vi "scan2D.vi"() -> ()   [LabVIEW 2019]
uses:
  National Instruments/LabVIEW 2019/instr.lib/Stanford Research 830/Public/Data/Read (All Parameters).vi
  National Instruments/LabVIEW 2019/instr.lib/Stanford Research 830/Stanford Research 830.lvlib
panel:
  in  "stop":bool
  in  "Tab Control":enum32{"Page 1", "Page 2", "Page 3"}(tab)
  out "progress":u8(slide) scale=0.0..100.0
  in  "Set zero":bool
  in  "Scanning range":T1
  in  "wait time":u32=3000
  in  "start":bool
  in  "file path (use dialog)":path
  in  "Cluster 2":T2={"Input Connection (0: Single-Ended Voltage) "=2, "Input Coupling (0: AC)"=0, "Input Notch Filter (0: None)"=0, "Input Shield Grounding (0: Float)"=1, "Internal Reference Frequency (1000 Hz)"=200.0, "Dynamic Reserve (-1: Auto Reserve)"=2, "Sensitivity (-1: Auto gain)"=16, "Time Constant (8: 100ms)"=10, "Low Pass Filter Slope (1: 12dB/oct)"=3, "Enable Sync Filter (F: Disable)"=FALSE, "save"=FALSE} {"Low Pass Filter Slope (1: 12dB/oct)" items=["6 dB/oct", "12 dB/oct", "18 db/oct", "24 dB/oct"]; "Time Constant (8: 100ms)" items=["10 us", "30 us", "100 us", "300 us", "1 ms", "3 ms", "10 ms", "30 ms", "100 ms", "300 ms", "1 s", "3 s", "10 s", "30 s", "100 s", "300 s", "1 ks", "3 ks", "10 ks", "30 ks"]; "Sensitivity (-1: Auto gain)" items=["Auto Gain"=-1, "2 nV/fA"=0, "5 nV/fA"=1, "10 nV/fA"=2, "20 nV/fA"=3, "50 nV/fA"=4, "100 nV/fA"=5, "200 nV/fA"=6, "500 nV/fA"=7, "1 uV/pA"=8, "2 uV/pA"=9, "5 uV/pA"=10, "10 uV/pA"=11, "20 uV/pA"=12, "50 uV/pA"=13, "100 uV/pA"=14, "200 uV/pA"=15, "500 uV/pA"=16, "1 mV/nA"=17, "2 mV/nA"=18, "5 mV/nA"=19, "10 mV/nA"=20, "20 mV/nA"=21, "50 mV/nA"=22, "100 mV/nA"=23, "200 mV/nA"=24, "500 mV/mA"=25, "1 V/uA"=26]; "Dynamic Reserve (-1: Auto Reserve)" items=["Auto Reserve"=-1, "High Reserve"=0, "Normal"=1, "Low Noise"=2]; "Input Shield Grounding (0: Float)" items=["Float", "Ground"]; "Input Notch Filter (0: None)" items=["None", "Line Notch", "2x Line Notch", "Both Notch Filters"]; "Input Coupling (0: AC)" items=["AC", "DC"]; "Input Connection (0: Single-Ended Voltage)" items=["Single-Ended Voltage", "Differential Voltage", "1 MOhm Current Gain", "100 MOhm Current Gain"]}
  in  "VISA resource name":refnum<visa-resource-name>="GPIB0::8::INSTR"
  out "error out":errorcluster
  out "Intensity Graph":dbl[][](graph)
  # "All relative position"
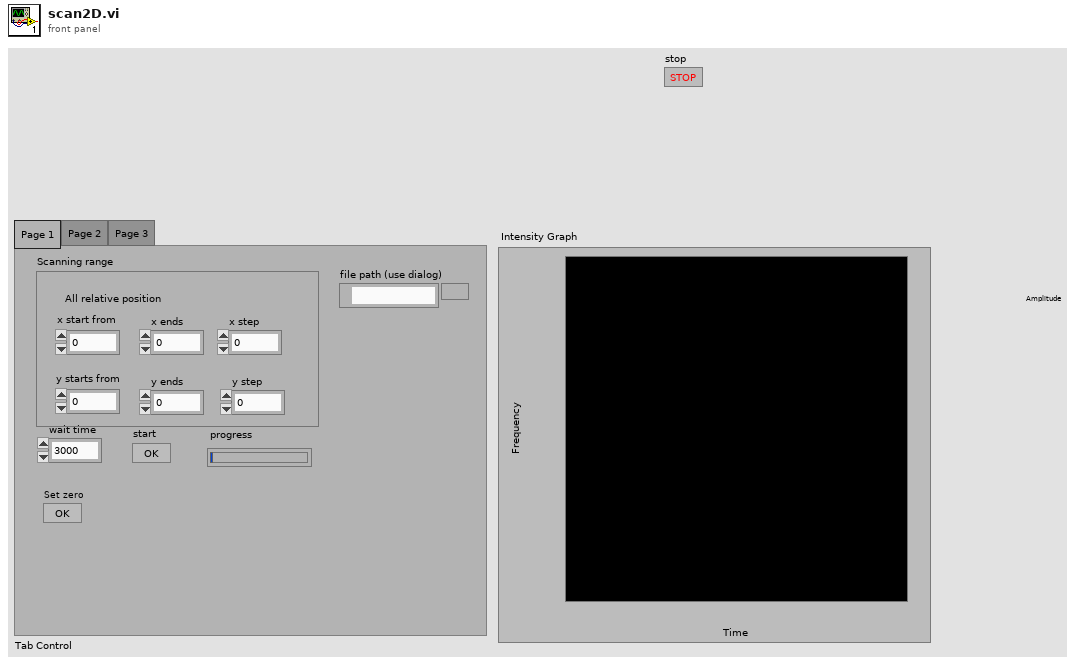
[diagram p1: front panel]
types:
  T1 = cluster{"x start from":dbl, "x ends":dbl, "x step":dbl, "y starts from":dbl, "y ends":dbl, "y step":dbl}
  T2 = cluster{"Input Connection (0: Single-Ended Voltage) ":u16, "Input Coupling (0: AC)":u16, "Input Notch Filter (0: None)":u16, "Input Shield Grounding (0: Float)":u16, "Internal Reference Frequency (1000 Hz)":dbl, "Dynamic Reserve (-1: Auto Reserve)":i16, "Sensitivity (-1: Auto gain)":i16, "Time Constant (8: 100ms)":u16, "Low Pass Filter Slope (1: 12dB/oct)":u16, "Enable Sync Filter (F: Disable)":bool, "save":bool}
  T3 = enum16{"open", "replace", "create", "open or create", "replace or create", "replace or create with confirmation"}
  T4 = cluster{"X-Value":dbl, "Y-Value":dbl, "R-Value":dbl, "Theta-Value":dbl, "Aux In 1 Value":dbl, "Aux In 2 Value":dbl, "Aux In 3 Value":dbl, "Aux In 4 Value":dbl, "Reference Frequency":dbl, "Channel 1 Display":dbl, "Channel 2 Display":dbl}
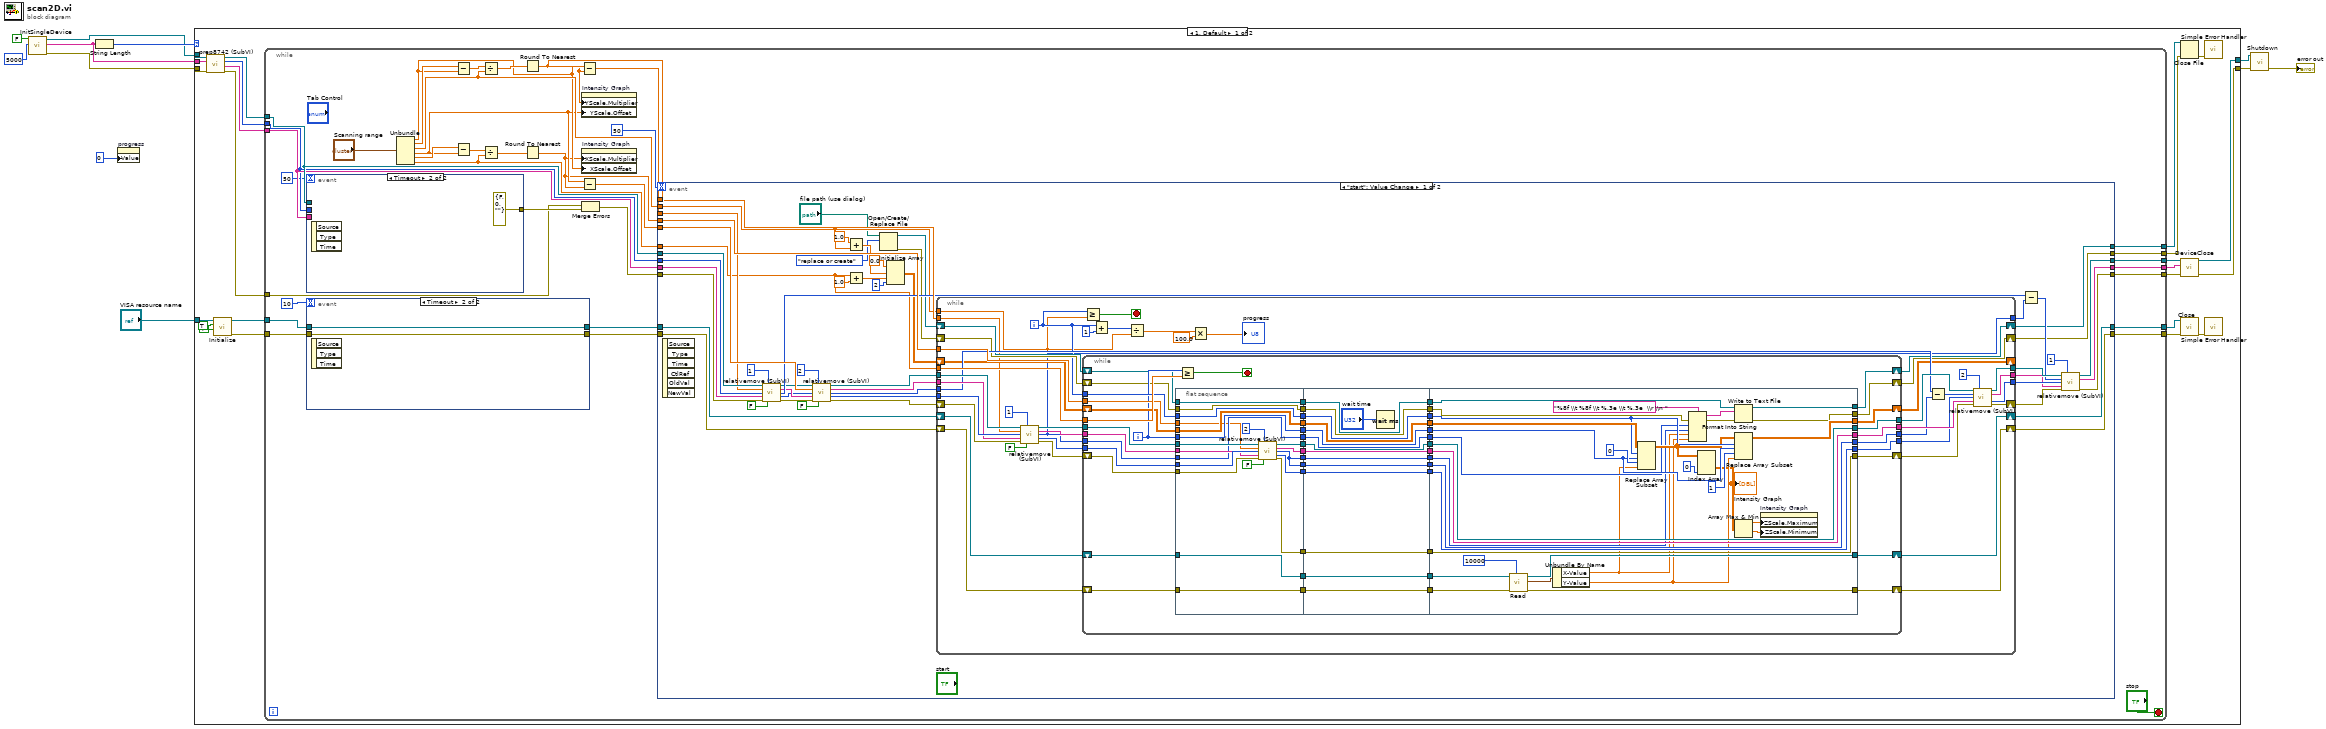
[diagram p0: block diagram]
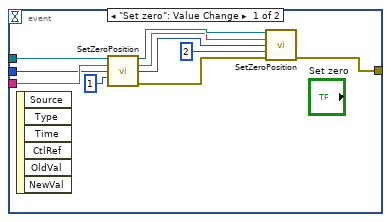
[diagram p2: hidden frame]
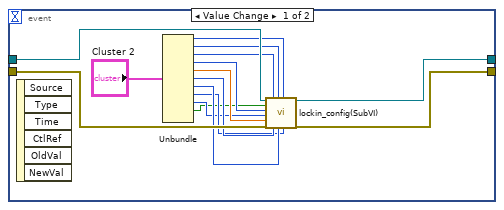
[diagram p3: hidden frame]
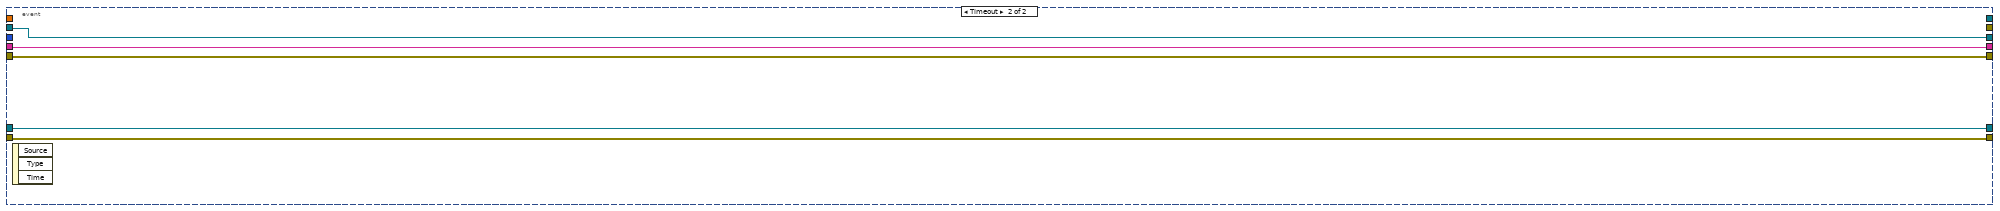
[diagram p4: hidden frame]
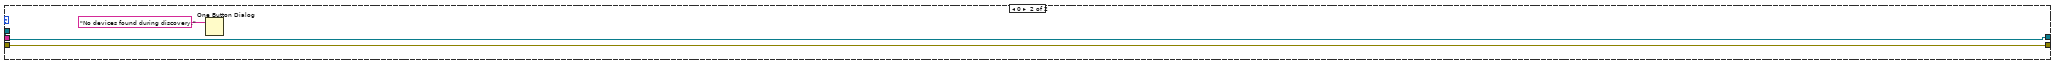
[diagram p5: hidden frame]
diagram:
  n1 = call "InitSingleDevice.vi"("msecDelayForDiscovery"=5000, "logging"=FALSE) -> ("error out"=w6:errorcluster, "DeviceKey Out"=w3:string, "CmdLib Out"=w4:refnum<k24>)  [unwired: 3 in]
  n2 = String Length(string=w3) -> (length=w9:i32)
  n3 = property on="progress" class="Slide (strict)"("Value"=u8 0 ("progress")) -> ()  [unwired: 2 in, 2 out]
  n4 = case shown="1, Default" w9 {
    tunnel: [w28 w321] -> w8
    tunnel: [w27 w320] -> w5
    tunnel: w6 -> [w34 w320]
    tunnel: w4 -> [w26 w321]
    tunnel: w3 -> [w25 _]
    tunnel: "VISA resource name" -> [w19 _]
    frame 1, Default {
      n5 = call "prep8742 (SubVI).vi"("error in (no error)"=w34, "DeviceKey Out in"=w25, ".NET Refnum in"=w26) -> ("error out"=w30:errorcluster, "DeviceKey Out out"=w31:string, "Device Address Out"=w32:i32, ".NET Refnum out"=w33:refnum<k24>)  [unwired: 4 in]
      n6 = call "Initialize.vi"("Reset (True)"=FALSE, "ID Query (True)"=TRUE, "VISA resource name"=w19) -> ("error out"=w22:errorcluster, "VISA resource name out"=w23:refnum<visa-resource-name>)  [unwired: 7 in]
      n7 = while {
        tunnel: w33 -> [w45]
        tunnel: w32 -> [w43]
        tunnel: w31 -> [w44]
        tunnel: w30 -> [w41]
        tunnel: [w53] -> w29
        tunnel: [w52] -> w24
        tunnel: w23 -> [w59]
        tunnel: w22 -> [w58]
        tunnel: [w55] -> w21
        tunnel: [w54] -> w20
        tunnel: [w50] -> w17
        tunnel: [w40] -> w14
        tunnel: [w39] -> w13
        stop <- "stop" stop-if-true
        n8 = event shown="[1] Timeout" {
          selector: _ -> [_ _]
          dyn-events: _ -> [_ _]
          timeout: 50 -> [_ _]
          tunnel: [w74 errorcluster {"status"=FALSE, "code"=0, "source"=""} ("error out")] -> w47
          tunnel: w45 -> [w73 _]
          tunnel: w44 -> [w72 _]
          tunnel: w43 -> [w71 _]
          event "Set zero": Value Change {
            n9 = event-data() -> ()  [unwired: 1 in, 6 out]
            n10 = call "SetZeroPosition.vi"("CmdLib In"=w73, "DeviceKey In"=w72, "Device Address In"=w71, "Motor"=1) -> ("CmdLib Out"=w80:refnum<k24>, "DeviceKey Out"=w79:string, "Device Address Out"=w78:i32, "error out"=w77:errorcluster)  [unwired: 8 in]
            n11 = call "SetZeroPosition.vi"("CmdLib In"=w80, "DeviceKey In"=w79, "Device Address In"=w78, "Motor"=2, "error in (no error)"=w77) -> ("error out"=w74:errorcluster)  [unwired: 7 in, 3 out]
          }
          event Timeout {
            n12 = event-data() -> ()  [unwired: 1 in, 3 out]
          }
        }
        n13 = event shown="[1] Timeout" {
          selector: _ -> [_ _]
          dyn-events: _ -> [_ _]
          timeout: 10 -> [_ _]
          tunnel: w59 -> [w96 w98]
          tunnel: w58 -> [w95 w97]
          tunnel: [w94 w98] -> w57
          tunnel: [w93 w97] -> w56
          event "Cluster 2.save": Value Change {
            n14 = event-data() -> ()  [unwired: 1 in, 6 out]
            n15 = Unbundle("Cluster 2") -> ("Input Connection (0: Single-Ended Voltage)"=w91:u16, "Input Coupling (0: AC)"=w90:u16, "Input Notch Filter (0: None)"=w89:u16, "Input Shield Grounding (0: Float)"=w87:u16, "Internal Reference Frequency (1000 Hz)"=w88:dbl, "Dynamic Reserve (-1: Auto Reserve)"=w86:i16, "Sensitivity (-1: Auto gain)"=w85:i16, "Time Constant (8: 100ms)"=w84:u16, "Low Pass Filter Slope (1: 12dB/oct)"=w83:u16, "Enable Sync Filter (F: Disable)"=w82:bool)  [unwired: 1 out]
            n16 = call "lockin_config(SubVI).vi"("VISA Refnum in"=w96, "Enable Sync Filter (F: Disable)"=w82, "Input Shield Grounding (0: Float)"=w87, "Low Pass Filter Slope (1: 12dB/oct)"=w83, "Internal Reference Frequency (1000 Hz)"=w88, "error in (no error)"=w95, "Input Notch Filter (0: None)"=w89, "Dynamic Reserve (-1: Auto Reserve)"=w86, "Input Coupling (0: AC)"=w90, "Sensitivity (-1: Auto gain)"=w85, "Input Connection (0: Single-Ended Voltage)"=w91, "Time Constant (8: 100ms)"=w84) -> ("VISA Refnum out"=w94:refnum<visa-resource-name>, "error out"=w93:errorcluster)  [unwired: 6 in]
          }
          event Timeout {
            n17 = event-data() -> ()  [unwired: 1 in, 3 out]
          }
        }
        n18 = Unbundle("Scanning range") -> ("x start from"=w38:dbl, "x ends"=w65:dbl, "x step"=w63:dbl, "y starts from"=w37:dbl, "y ends"=w64:dbl, "y step"=w49:dbl)
        n19 = Subtract(x=w65, y=w38) -> (x-y=w69:dbl)
        n20 = Subtract(x=w64, y=w37) -> (x-y=w67:dbl)
        n21 = Divide(x=w69, y=w63) -> (x/y=w68:dbl)
        n22 = Divide(x=w67, y=w49) -> (x/y=w66:dbl)
        n23 = Round To Nearest(number=w68) -> (nearest integer value=w35:dbl)
        n24 = Round To Nearest(number=w66) -> (nearest integer value=w36:dbl)
        n25 = Subtract(x=w38, y=w35) -> (x-y=w60:dbl)
        n26 = Subtract(x=w37, y=w36) -> (x-y=w61:dbl)
        n27 = property on="Intensity Graph" class="IntGraph (strict)"("YScale.Multiplier"=w35, "YScale.Offset"=w37) -> ()  [unwired: 2 in, 2 out]
        n28 = property on="Intensity Graph" class="IntGraph (strict)"("XScale.Multiplier"=w36, "XScale.Offset"=w38) -> ()  [unwired: 2 in, 2 out]
        n29 = Merge Errors(w41, w47) -> (w46:errorcluster)
        n30 = event shown="[0] \"start\": Value Change" {
          selector: _ -> [_ _]
          dyn-events: _ -> [_ _]
          timeout: 50 -> [_ _]
          tunnel: w63 -> [w113 _]
          tunnel: w45 -> [w149 w315]
          tunnel: w43 -> [w148 _]
          tunnel: w44 -> [w147 w316]
          tunnel: w46 -> [w146 w317]
          tunnel: w36 -> [w145 _]
          tunnel: w61 -> [w144 _]
          tunnel: w35 -> [w143 _]
          tunnel: w60 -> [w142 _]
          tunnel: w57 -> [w141 w318]
          tunnel: w56 -> [w140 w319]
          tunnel: [w110 w318] -> w55
          tunnel: [w139 w319] -> w54
          tunnel: [w138 w315] -> w53
          tunnel: [w137 w316] -> w52
          tunnel: [w136 w317] -> w50
          tunnel: w49 -> [w99 _]
          tunnel: [w100 _] -> w39
          tunnel: [w101 _] -> w40
          event "start": Value Change {
            n31 = event-data() -> ()  [unwired: 1 in, 6 out]
            n32 = call "relativemove (SubVI).vi"(".NET Refnum in"=w149, "Motor Number"=1, "Relative Steps"=w142, "Device Address In"=w148, "DeviceKey In"=w147, "error in (no error)"=w146, "stop"=FALSE) -> (".NET Refnum out"=w134:refnum<k24>, "DeviceKey Out"=w133:string, "Position"=w135:i32, "Device Address Out"=w132:i32, "error out"=w131:errorcluster)  [unwired: 4 in]
            n33 = call "relativemove (SubVI).vi"(".NET Refnum in"=w134, "Motor Number"=2, "Relative Steps"=w144, "Device Address In"=w132, "DeviceKey In"=w133, "error in (no error)"=w131, "stop"=FALSE) -> (".NET Refnum out"=w126:refnum<k24>, "DeviceKey Out"=w125:string, "Position"=w122:i32, "Device Address Out"=w127:i32, "error out"=w128:errorcluster)  [unwired: 4 in]
            n34 = Add(x=1.0, y=w113) -> (x+y=w107:dbl)
            n35 = Add(x=w99, y=1.0) -> (x+y=w109:dbl)
            n36 = Open/Create/Replace File(file path (use dialog)="file path (use dialog)", operation (0:open)=T3."replace or create") -> (refnum out=w103:refnum<file>, error out=w102:errorcluster)  [unwired: 4 in, 1 out]
            n37 = Initialize Array(0.0 ("element"), w107, w109, 2 ("dimension size")) -> (w112:dbl[][][])
            n38 = while {
              tunnel: [w173] -> w120
              tunnel: w143 -> [w152]
              tunnel: w145 -> [w193]
              tunnel: w113 -> [w150]
              tunnel: w99 -> [w183]
              tunnel: w127 -> [w191]
              tunnel: w126 -> [w190]
              tunnel: w125 -> [w189]
              tunnel: [w174] -> w116
              shift-right: [w175] -> w115
              shift-left: w128 -> [w192]
              tunnel: w122 -> [w176]
              tunnel: [w171] -> w117
              tunnel: [w154] -> w121
              shift-right: [w168] -> w139
              shift-left: w140 -> [w169]
              shift-right: [w166] -> _
              shift-left: w112 -> [w167]
              shift-right: [w165] -> w110
              shift-left: w141 -> [w170]
              shift-right: [w162] -> w101
              shift-left: w102 -> [w163]
              shift-right: [w153] -> w100
              shift-left: w103 -> [w164]
              i -> [w160]
              stop <- w151 stop-if-true
              n39 = call "relativemove (SubVI).vi"(".NET Refnum in"=w190, "Motor Number"=1, "Relative Steps"=w152, "Device Address In"=w191, "DeviceKey In"=w189, "error in (no error)"=w192, "stop"=FALSE) -> (".NET Refnum out"=w187:refnum<k24>, "DeviceKey Out"=w186:string, "Position"=w154:i32, "Device Address Out"=w185:i32, "error out"=w184:errorcluster)  [unwired: 4 in]
              n40 = while {
                tunnel: [w240] -> w181
                tunnel: w193 -> [w245]
                tunnel: w187 -> [w241]
                tunnel: w186 -> [w242]
                tunnel: w185 -> [w243]
                tunnel: [w239] -> w180
                tunnel: w183 -> [w246]
                shift-right: [w237] -> w178
                shift-left: w184 -> [w244]
                tunnel: [w238] -> w179
                shift-right: [w236] -> w168
                shift-left: w169 -> [w234]
                tunnel: w160 -> [w218]
                shift-right: [w212] -> w166
                shift-left: w167 -> [w219]
                shift-right: [w211] -> w165
                shift-left: w170 -> [w235]
                shift-right: [w204] -> w162
                shift-left: w163 -> [w205]
                tunnel: [w203] -> w155
                tunnel: w154 -> [w200]
                shift-right: [w195] -> w153
                shift-left: w164 -> [w208]
                i -> [w213]
                stop <- w194 stop-if-true
                n41 = flat-sequence {
                  tunnel: w245 -> [w247]
                  tunnel: w244 -> [w264]
                  tunnel: w243 -> [w263]
                  tunnel: w242 -> [w262]
                  tunnel: w241 -> [w261]
                  tunnel: [w260] -> w233
                  tunnel: [w259] -> w231
                  tunnel: [w258] -> w229
                  tunnel: [w257] -> w227
                  tunnel: [w256] -> w225
                  tunnel: w235 -> [w256]
                  tunnel: [w255] -> w223
                  tunnel: w234 -> [w255]
                  tunnel: [w254] -> w220
                  tunnel: w219 -> [w254]
                  tunnel: w218 -> [w253]
                  tunnel: [w253] -> w217
                  tunnel: [w252] -> w214
                  tunnel: w213 -> [w252]
                  tunnel: [w251] -> w209
                  tunnel: w208 -> [w251]
                  tunnel: [w250] -> w206
                  tunnel: w205 -> [w250]
                  tunnel: [w248] -> w201
                  tunnel: w200 -> [w249]
                  tunnel: [w249] -> w199
                  tunnel: [w248] -> w197
                  tunnel: w233 -> [w281]
                  tunnel: [w281] -> w232
                  tunnel: w231 -> [w280]
                  tunnel: [w280] -> w230
                  tunnel: w229 -> [w279]
                  tunnel: [w279] -> w228
                  tunnel: w227 -> [w278]
                  tunnel: [w278] -> w226
                  tunnel: w225 -> [w277]
                  tunnel: [w277] -> w224
                  tunnel: w223 -> [w276]
                  tunnel: [w276] -> w222
                  tunnel: [w274] -> w221
                  tunnel: w220 -> [w274]
                  tunnel: w217 -> [w273]
                  tunnel: [w273] -> w216
                  tunnel: [w272] -> w215
                  tunnel: w214 -> [w272]
                  tunnel: [w271] -> w210
                  tunnel: w209 -> [w271]
                  tunnel: [w270] -> w207
                  tunnel: w206 -> [w270]
                  tunnel: [w269] -> w202
                  tunnel: w201 -> [w269]
                  tunnel: w199 -> [w268]
                  tunnel: [w268] -> w198
                  tunnel: w197 -> [w267]
                  tunnel: [w267] -> w196
                  tunnel: [w314] -> w240
                  tunnel: w232 -> [w314]
                  tunnel: [w313] -> w239
                  tunnel: w230 -> [w313]
                  tunnel: [w312] -> w238
                  tunnel: w228 -> [w312]
                  tunnel: [w311] -> w237
                  tunnel: w226 -> [w311]
                  tunnel: [w308] -> w236
                  tunnel: [w307] -> w211
                  tunnel: w224 -> [w306]
                  tunnel: w222 -> [w305]
                  tunnel: w221 -> [w304]
                  tunnel: w216 -> [w302]
                  tunnel: w215 -> [w301]
                  tunnel: [w297] -> w212
                  tunnel: w210 -> [w296]
                  tunnel: w207 -> [w287]
                  tunnel: [w295] -> w195
                  tunnel: [w294] -> w204
                  tunnel: [w293] -> w203
                  tunnel: w202 -> [w293]
                  tunnel: w198 -> [w291]
                  tunnel: w196 -> [w290]
                  frame #0 {
                    n42 = call "relativemove (SubVI).vi"(".NET Refnum in"=w261, "Motor Number"=2, "Relative Steps"=w247, "Device Address In"=w263, "DeviceKey In"=w262, "error in (no error)"=w264, "stop"=FALSE) -> (".NET Refnum out"=w260:refnum<k24>, "DeviceKey Out"=w259:string, "Position"=w248:i32, "Device Address Out"=w258:i32, "error out"=w257:errorcluster)  [unwired: 4 in]
                  }
                  frame #1 {
                    n43 = Wait (ms)(milliseconds to wait="wait time") -> ()  [unwired: 1 out]
                  }
                  frame #2 {
                    n44 = call-poly "Read.vi"("Timeout (10000 ms)"=u32 10000, "error in (no error)"=w305, "VISA resource name"=w306) -> ("error out"=w308:errorcluster, "Parameter Values"=w310:T4, "VISA resource name out"=w307:refnum<visa-resource-name>)  [unwired: 6 in]
                    n45 = Unbundle By Name(w310) -> ("X-Value"=w285:dbl, "Y-Value"=w289:dbl)
                    n46 = Replace Array Subset(array=w304, new element=w285, index (dim 0)=w302, index (dim 1)=w301, index (dim 2)=0 ("disabled index (col)")) -> (w299:dbl[][][])
                    n47 = Format Into String(format string="%8f \\t %8f \\t %.3e \\t %.3e  \\r \\n ", error in=w287, w291, w290, w285, w289) -> (resulting string=w288:string, error out=w286:errorcluster)  [unwired: 1 in]
                    n48 = Index Array(array=w299, index (dim 2)=0 ("index")) -> (element=w284:dbl[][])  [unwired: 2 in]
                    "Intensity Graph" <- w284
                    n49 = Write to Text File(file (use dialog)=w296, text=w288, error in=w286) -> (refnum out=w295:refnum<file>, error out=w294:errorcluster)  [unwired: 1 in, 1 out]
                    n50 = Replace Array Subset(array=w299, new element=w289, index (dim 0)=w302, index (dim 1)=w301, index (dim 2)=1 ("disabled index (col)")) -> (w297:dbl[][][])
                    n51 = Array Max & Min(array=w284) -> (max value=w283:dbl, min value=w282:dbl)  [unwired: 2 out]
                    n52 = property on="Intensity Graph" class="IntGraph (strict)"("ZScale.Maximum"=w283, "ZScale.Minimum"=w282) -> ()  [unwired: 2 in, 2 out]
                  }
                }
                n53 = Greater Or Equal?(x=w213, y=w246) -> (x >= y?=w194:bool)
              }
              n54 = Greater Or Equal?(x=w160, y=w150) -> (x >= y?=w151:bool)
              n55 = Add(x=w160, y=1) -> (x+y=w159:i32)
              n56 = Divide(x=w159, y=w150) -> (x/y=w161:dbl)
              n57 = Multiply(x=w161, y=100.0) -> (x*y=→"progress":dbl)
              n58 = Subtract(x=w176, y=w155) -> (x-y=w177:i32)
              n59 = call "relativemove (SubVI).vi"(".NET Refnum in"=w181, "Motor Number"=2, "Relative Steps"=w177, "Device Address In"=w179, "DeviceKey In"=w180, "error in (no error)"=w178) -> (".NET Refnum out"=w173:refnum<k24>, "DeviceKey Out"=w174:string, "Device Address Out"=w171:i32, "error out"=w175:errorcluster)  [unwired: 5 in, 1 out]
            }
            n60 = Subtract(x=w135, y=w121) -> (x-y=w118:i32)
            n61 = call "relativemove (SubVI).vi"(".NET Refnum in"=w120, "Motor Number"=1, "Relative Steps"=w118, "Device Address In"=w117, "DeviceKey In"=w116, "error in (no error)"=w115) -> (".NET Refnum out"=w138:refnum<k24>, "DeviceKey Out"=w137:string, "error out"=w136:errorcluster)  [unwired: 5 in, 2 out]
          }
          event Timeout {
            n62 = event-data() -> ()  [unwired: 1 in, 3 out]
          }
        }
      }
      n63 = Close File(refnum=w13, error in=w14) -> (error out=w15:errorcluster)  [unwired: 1 out]
      n64 = call "DeviceClose.vi"("error in (no error)"=w17, "DeviceKey In"=w24, "CmdLib In"=w29) -> ("error out"=w27:errorcluster, "CmdLib Out"=w28:refnum<k24>)  [unwired: 2 in, 1 out]
      n65 = call "Close.vi"("error in (no error)"=w20, "VISA resource name"=w21) -> ("error out"=w18:errorcluster)  [unwired: 9 in]
      n66 = call <vilib>:"Simple Error Handler.vi"("error in (no error)"=w15) -> ()  [unwired: 4 in, 5 out]
      n67 = call <vilib>:"Simple Error Handler.vi"("error in (no error)"=w18) -> ()  [unwired: 4 in, 5 out]
    }
    frame 0 {
      n68 = One Button Dialog(message="No devices found during discovery.") -> ()  [unwired: 1 in, 1 out]
    }
  }
  n69 = call "Shutdown.vi"("error in (no error)"=w5, "CmdLib In"=w8) -> ("error out"=→"error out":errorcluster)  [unwired: 4 in, 1 out]
